vi "8-Axis (Manual).vi"() -> ()   [LabVIEW 2014]
uses:
  EMC API/EMC_Typedef_Motor_Parameters.ctl
  Typedef/Typedef_Motor_Action.ctl
  <vilib>/Motion/Express/_s/nimc.ex.power.power.axis.vi
  <vilib>/Motion/Express/_s/nimc.ex.resetPosition.resetPosition.axis.vi
  <vilib>/Motion/Express/_s/nimc.ex.findReferenceMove.startReferenceMove.axis.modeReverseLimit.vi
  <vilib>/Motion/Express/_s/nimc.ex.findReferenceMove.startReferenceMove.axis.modeHome.vi
  <vilib>/Motion/Express/_s/nimc.ex.findReferenceMove.startReferenceMove.axis.modeForwardLimit.vi
  <vilib>/Motion/Express/_s/nimc.ex.read.readTrajectoryData.axis.vi
  <vilib>/Motion/Express/_s/nimc.ex.read.readMotionIO.axis.vi
  <vilib>/Motion/BlockNode/FB.NIMotion.xnode
  Functional_Global/Typedef_FPGA_Interface_Action.ctl
  <vilib>/Motion/Express/_s/nimc.ex.clearFaults.clearFaults.axis.vi
panel:
  in  "velocity":dbl=1000.0
  in  "position[]":dbl[](array[numeric])=[5000.0, 5000.0, 5000.0, 5000.0, 5000.0, 5000.0, 5000.0, 5000.0]
  in  "resource":refnum<k21>="Axis 1"
  out "home active":bool
  out "rev. limit active":bool
  out "fwd. limit active":bool
  out "XY Graph":cluster{"X Array":dbl[], "Y Array":dbl[]}(graph)
  in  "interval":dbl=0.01 format="%#_13g"
  in  "Gear in/out":enum16{"Gear in", "Gear out"}(ring)
  in  "denominator":i32=1
  in  "numerator":i32=1
  in  "Master Axis":T1(ring)
  out "Array":dbl[](array[knob]) scale=0.0..1600.0
  in  "Clear Errors":bool
  in  "Command":T2
  in  "Motion Parameters":T3={"position"=1000.0, "velocity"=1000.0, "acceleration"=10000.0, "deceleration"=10000.0, "accel. jerk"=10000.0, "decel. jerk"=10000.0}
  in  "Axis Index":T1(ring)
  out "error":errorcluster
  out "Numeric":i32
  in  "Stop all motors":bool
  in  "Execute Command":bool
  in  "stop":bool
  out "Axis Velocities":T4(graph)
  out "Axis Positions":T4(graph)
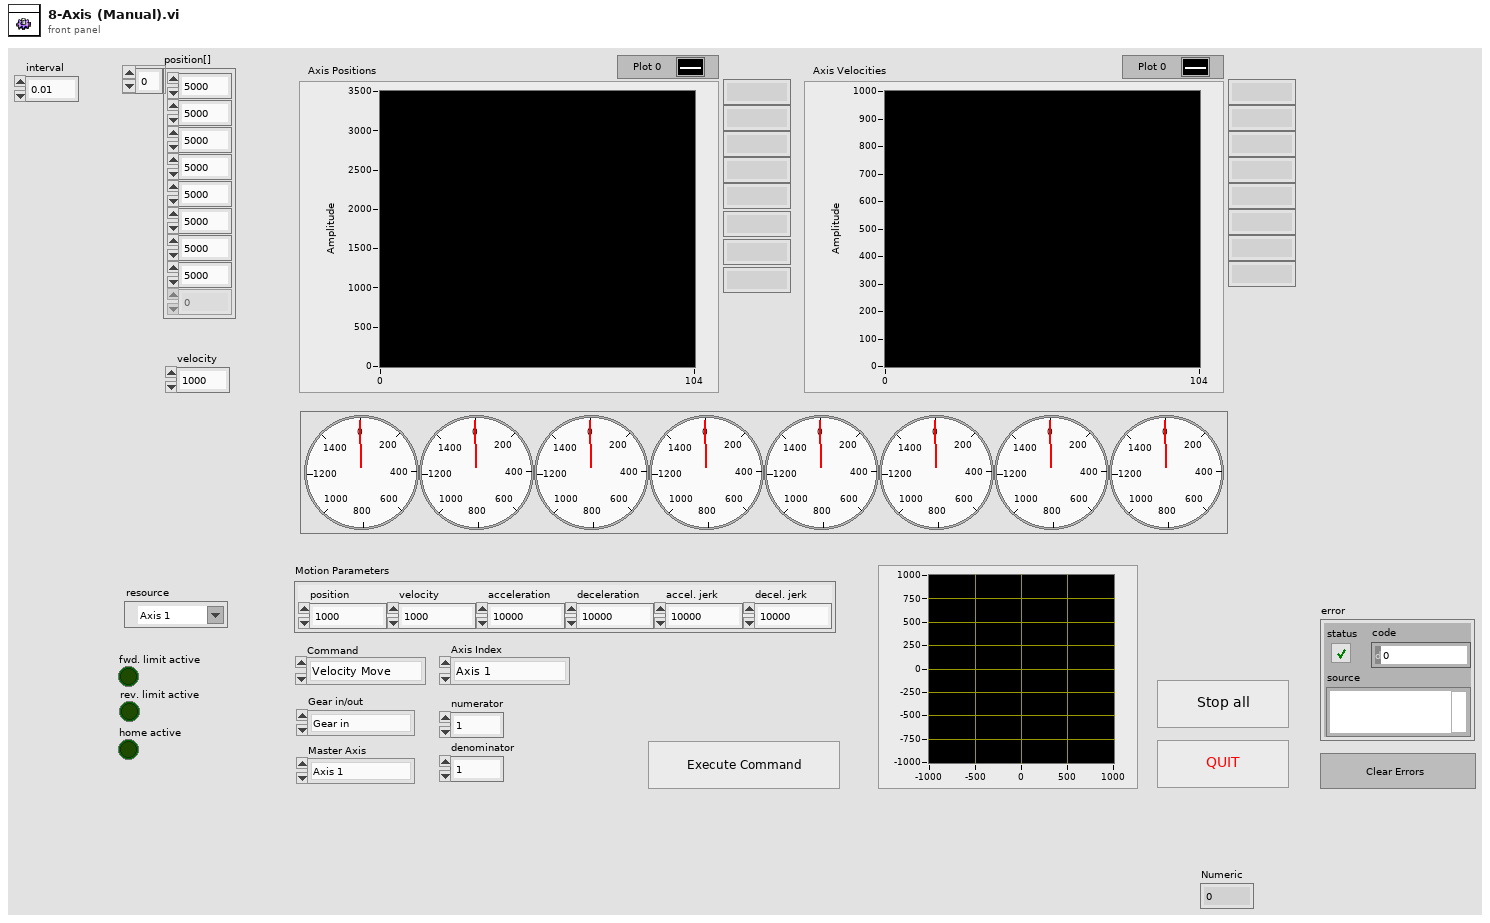
[diagram p1: front panel]
types:
  T1 = enum16{"Axis 1", "Axis 2", "Axis 3", "Axis 4", "Axis 5", "Axis 6", "Axis 7", "Axis 8"}
  T2 = typedef "Typedef_Motor_Action.ctl" = enum16{"Velocity Move", "REL Pos Move", "ABS Pos Move", "Stop", "Reset Position", "Coordinate_move", "Contour_move", "Gearing", "Find Fwd Limit", "Find Rev Limit", "Find Home"}
  T3 = typedef "EMC_Typedef_Motor_Parameters.ctl" = cluster{"position":dbl, "velocity":dbl, "acceleration":dbl, "deceleration":dbl, "accel. jerk":dbl, "decel. jerk":dbl}
  T4 = cluster{"[0]":dbl, "[1]":dbl, "[2]":dbl, "[3]":dbl, "[4]":dbl, "[5]":dbl, "[6]":dbl, "[7]":dbl}
  T5 = typedef "Typedef_FPGA_Interface_Action.ctl" = enum16{"Initialize FPGA", "Get FPGA Reference", "Close FPGA"}
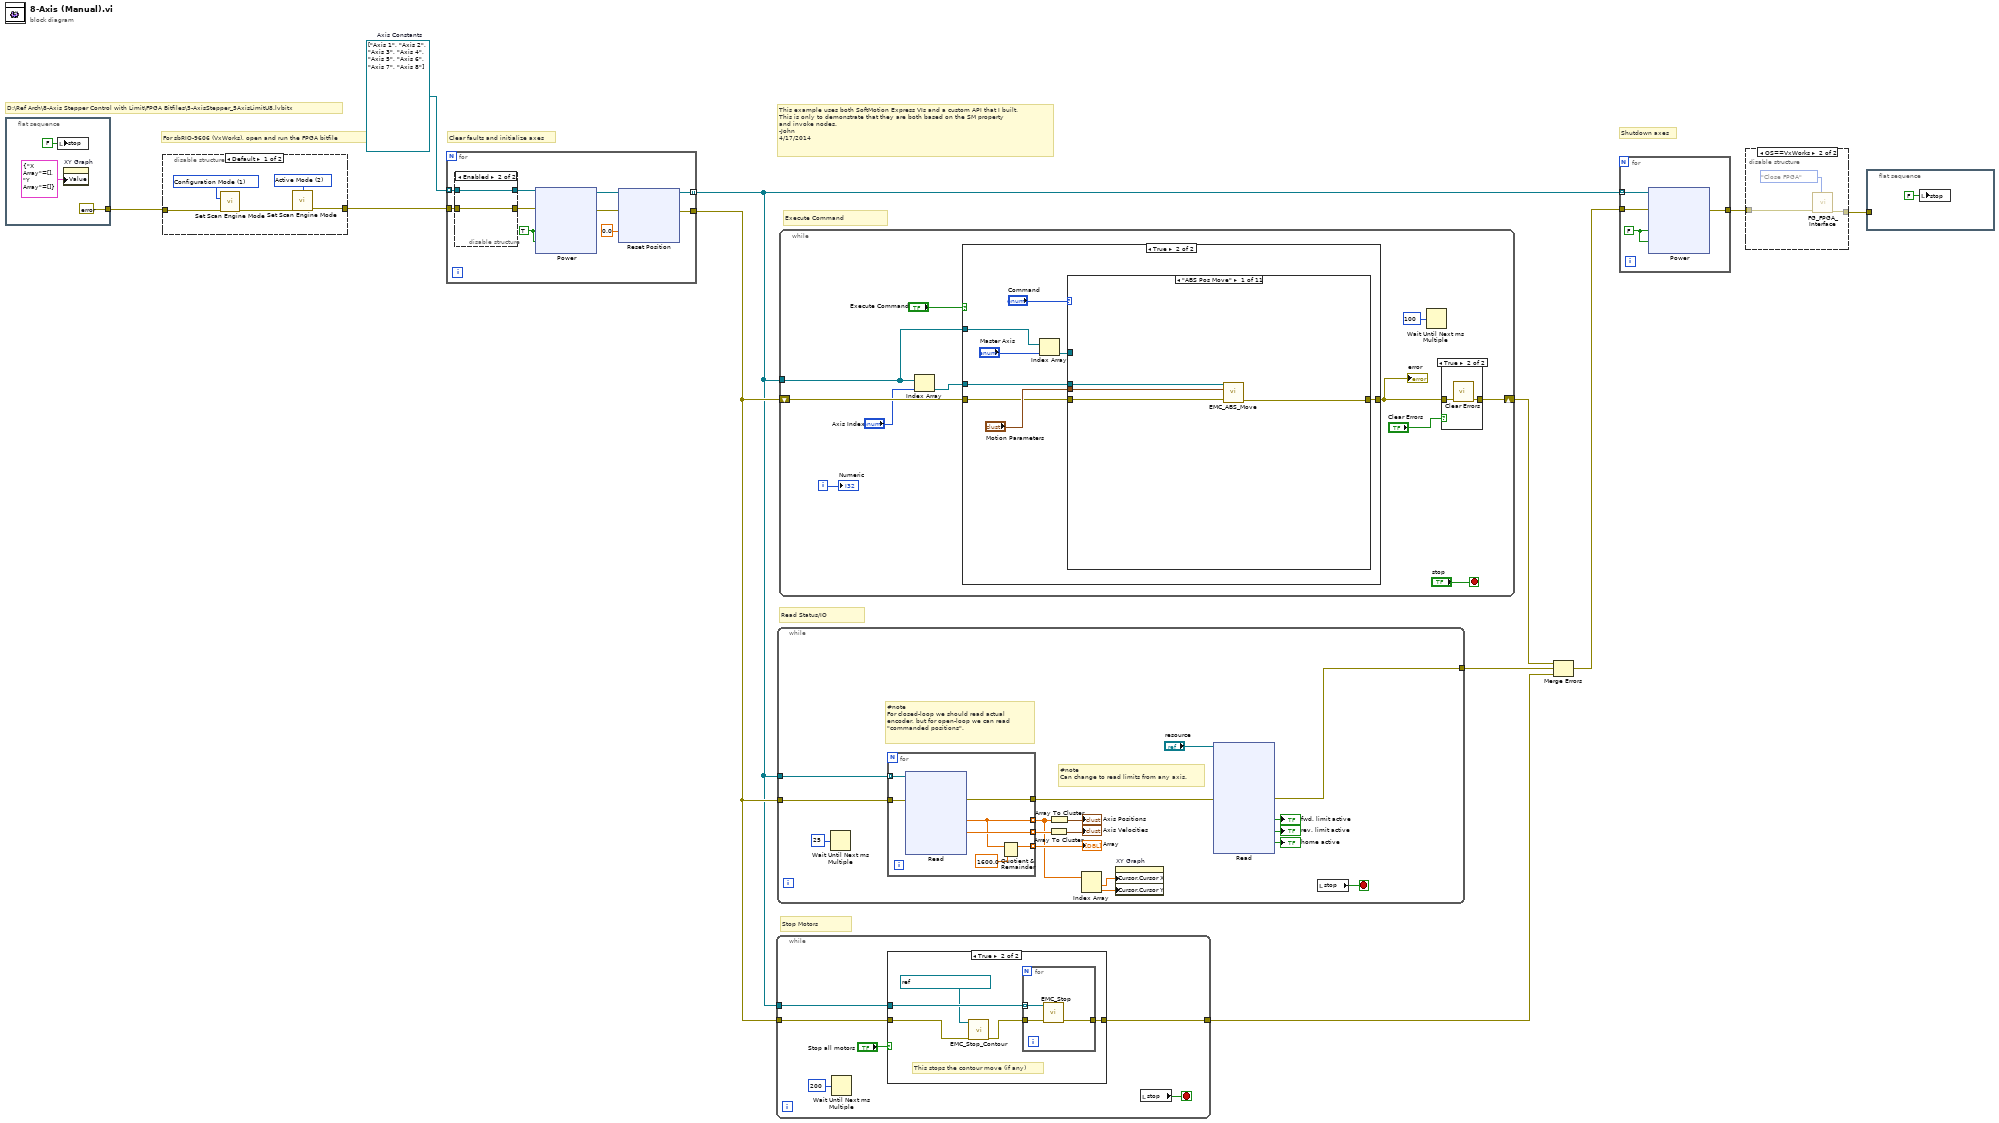
[diagram p0: block diagram]
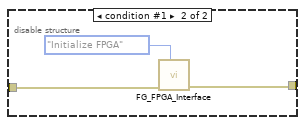
[diagram p3: hidden frame]
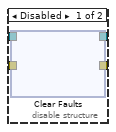
[diagram p4: hidden frame]
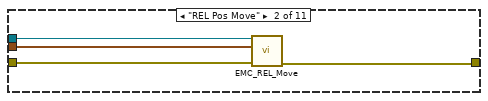
[diagram p8: hidden frame]
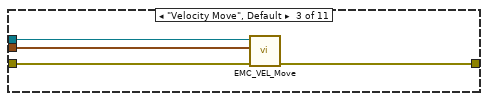
[diagram p9: hidden frame]
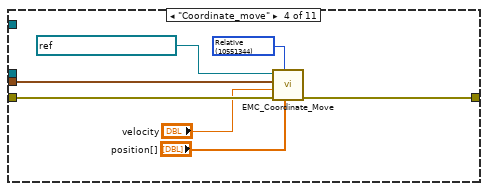
[diagram p10: hidden frame]
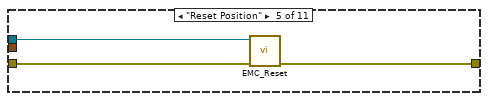
[diagram p11: hidden frame]
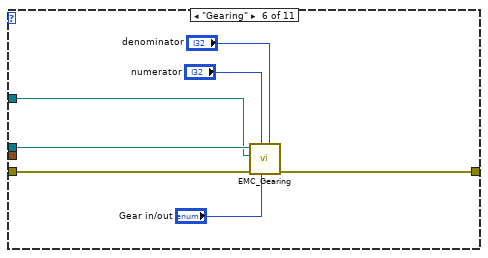
[diagram p12: hidden frame]
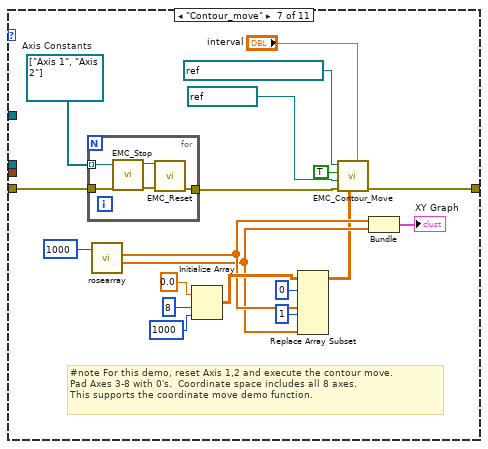
[diagram p13: hidden frame]
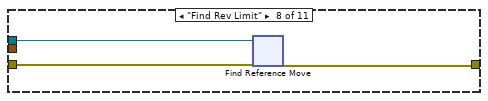
[diagram p14: hidden frame]
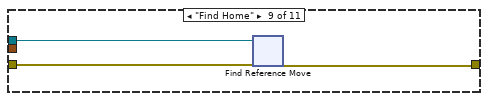
[diagram p15: hidden frame]
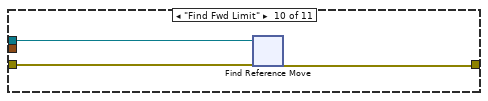
[diagram p16: hidden frame]
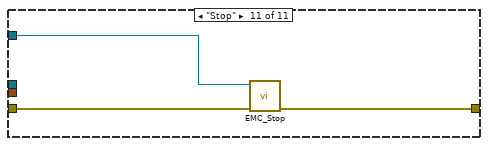
[diagram p17: hidden frame]
diagram:
  w10 = refnum<k21>[] ["Axis 1", "Axis 2", "Axis 3", "Axis 4", "Axis 5", "Axis 6", "Axis 7", "Axis 8"]  # Axis Constants
  # "For sbRIO-9606 (VxWorks), open and run the FPGA bitfile"
  # "D:\\Ref Arch\\8-Axis Stepper Control with Limit\\FPGA Bitfiles\\5-AxisStepper_5AxisLimitU8.lvbitx"
  # "Clear faults and initialize axes"
  # "This example uses both SoftMotion Express VIs and a custom API that I built.\nThis is only to demonstrate that they are both based on the SM property\nand invoke nodes. \n-John\n4/17/2014"
  # "Shutdown axes"
  # "Execute Command"
  # "Read Status/IO"
  # "Stop Motors"
  n1 = flat-sequence {
    tunnel: [errorcluster {"status"=FALSE, "code"=0, "source"=""} ("error in (no error)")] -> w7
    frame #0 {
      n2 = local write "stop"(FALSE ("stop")) -> ()
      n3 = property on="XY Graph" class="XYGraph (strict)"("Value"=cluster{"X Array":dbl[], "Y Array":dbl[]} {"X Array"=[], "Y Array"=[]} ("XY Graph")) -> ()  [unwired: 2 in, 2 out]
    }
  }
  n4 = disable-structure shown="Default" {
    disable-tunnel: [w19 w20] -> w4
    disable-tunnel: w7 -> [w18 w21]
    frame condition #0 (active) {
      w15 = 1 items=["Configuration Mode"=1, "Active Mode"=2] ("mode (Active Mode)")
      w16 = 2 items=["Configuration Mode"=1, "Active Mode"=2] ("mode (Active Mode)")
      n5 = call <vilib>:"Set Scan Engine Mode.vi"("mode (Active Mode)"=w15, "error in (no error)"=w18) -> ("error out"=w17:errorcluster)  [unwired: 13 in]
      n6 = call <vilib>:"Set Scan Engine Mode.vi"("mode (Active Mode)"=w16, "error in (no error)"=w17) -> ("error out"=w19:errorcluster)  [unwired: 13 in]
    }
    frame condition #1 {
      n7 = call "FG_FPGA_Interface.vi"("Action"=Typedef_FPGA_Interface_Action."Initialize FPGA", "error in"=w21) -> ("error out"=w20:errorcluster)  [unwired: 9 in]
    }
  }
  n8 = for {
    tunnel: w10 -> [w26] mode=indexing
    tunnel: w4 -> [w25]
    tunnel: [w28] -> w3
    tunnel: [w27] -> w1 mode=indexing
    w32 = TRUE ("enable axis")
    n9 = disable-structure shown="Enabled" {
      disable-tunnel: w26 -> [w36 w42]
      disable-tunnel: w25 -> [w35 w41]
      disable-tunnel: [w34 w42] -> w24
      disable-tunnel: [w33 w41] -> w23
      frame Disabled {
        n10 = xnode ("Clear Faults")("resource"=w36, "error in"=w35) -> ("resource out"=w34:refnum<k21>, "error out"=w33:errorcluster)
      }
      frame Enabled {
      }
    }
    n11 = xnode ("Power")("enable axis"=w32, "enable drive"=w32, "resource"=w24, "error in"=w23) -> ("resource out"=w31:refnum<k21>, "error out"=w30:errorcluster)
    n12 = xnode ("Reset Position")("position"=0.0, "resource"=w31, "error in"=w30) -> ("resource out"=w27:refnum<k21>, "error out"=w28:errorcluster)
  }
  n13 = while {
    tunnel: w3 -> [w62]
    tunnel: w1 -> [w60]
    tunnel: [w58] -> w11
    stop <- w63 stop-if-true
    n14 = Wait Until Next ms Multiple(millisecond multiple=u32 200) -> ()  [unwired: 1 out]
    n15 = case shown="True" "Stop all motors" {
      tunnel: w62 -> [w64 w67]
      tunnel: [w64 w69] -> w58
      tunnel: w60 -> [_ w68]
      frame False {
      }
      frame True {
        # "This stops the contour move (if any)"
        n16 = call "EMC_Stop_Contour.vi"("error in (no error)"=w67, "coordinate"=refnum<k21> "Coordinate Space 1") -> ("error out"=w65:errorcluster)  [unwired: 9 in]
        n17 = for {
          tunnel: w65 -> [w72]
          tunnel: w68 -> [w70] mode=indexing
          tunnel: [w71] -> w69
          n18 = call "EMC_Stop.vi"("error in (no error)"=w72, "axis"=w70) -> ("error out"=w71:errorcluster)  [unwired: 8 in, 1 out]
        }
      }
    }
    n19 = local read "stop"() -> (w63:bool)
  }
  n20 = while {
    tunnel: w3 -> [w85]
    tunnel: w1 -> [w84]
    tunnel: [w73] -> w9
    stop <- w89 stop-if-true
    # "#note \nCan change to read limits from any axis."
    # "#note \nFor closed-loop we should read actual \nencoder, but for open-loop we can read\n\"commanded positions\"."
    n21 = Wait Until Next ms Multiple(millisecond multiple=u32 25) -> ()  [unwired: 1 out]
    n22 = for {
      tunnel: [w124] -> w75
      tunnel: [w119] -> w82 mode=indexing
      tunnel: [w123] -> w88 mode=indexing
      tunnel: w85 -> [w122]
      tunnel: w84 -> [w121] mode=indexing
      tunnel: [w118] -> w83 mode=indexing
      n23 = xnode ("Read")("resource"=w121, "error in"=w122) -> ("commanded position"=w119:dbl, "commanded vel."=w123:dbl, "error out"=w124:errorcluster)  [unwired: 2 out]
      n24 = Quotient & Remainder(x=w119, y=1600.0) -> (x-y*floor(x/y)=w118:dbl)  [unwired: 1 out]
    }
    "Array" <- w83
    n25 = Array To Cluster(array=w88) -> (cluster=→"Axis Velocities":T4)
    n26 = Array To Cluster(array=w82) -> (cluster=→"Axis Positions":T4)
    n27 = Index Array(array=w82) -> (element #1=w81:dbl, element #2=w80:dbl)  [unwired: 2 in]
    n28 = property on="XY Graph" class="XYGraph (strict)"("Cursor.Cursor X"=w81, "Cursor.Cursor Y"=w80) -> ()  [unwired: 2 in, 2 out]
    n29 = xnode ("Read")("resource"="resource", "error in"=w75) -> ("fwd. limit active"=→"fwd. limit active":bool, "rev. limit active"=→"rev. limit active":bool, "home active"=→"home active":bool, "error out"=w73:errorcluster)  [unwired: 6 out]
    n30 = local read "stop"() -> (w89:bool)
  }
  n31 = while {
    tunnel: w1 -> [w132]
    shift-right: [w133] -> w6
    shift-left: w3 -> [w137]
    i -> [w142]
    stop <- "stop" stop-if-true
    n32 = Index Array(array=w132, index="Axis Index") -> (element=w138:refnum<k21>)
    n33 = case shown="True" "Execute Command" {
      tunnel: w137 -> [w146 w153]
      tunnel: w138 -> [_ w152]
      tunnel: [w146 w151] -> w134
      tunnel: w132 -> [_ w148]
      frame False {
      }
      frame True {
        n34 = Index Array(array=w148, index="Master Axis") -> (element=w147:refnum<k21>)
        n35 = case shown="\"ABS Pos Move\"" "Command" {
          tunnel: "Motion Parameters" -> [w155 w159 w166 w167 _ _ _ _ _ _ _]
          tunnel: w153 -> [w158 w162 w165 w173 w176 w183 w195 w209 w228 w249 w269]
          tunnel: w152 -> [w156 w160 w164 _ w175 w182 _ w208 w227 w248 _]
          tunnel: [w157 w161 w163 w172 w174 w181 w202 w210 w229 w250 w268] -> w151
          tunnel: w147 -> [_ _ _ _ _ w177 _ _ _ _ w267]
          frame "ABS Pos Move" {
            n36 = call "EMC_ABS_Move.vi"("error in (no error)"=w158, "Motion Parameters"=w155, "axis"=w156) -> ("error out"=w157:errorcluster)  [unwired: 8 in]
          }
          frame "REL Pos Move" {
            n37 = call "EMC_REL_Move.vi"("error in (no error)"=w162, "Motion Parameters"=w159, "axis"=w160) -> ("error out"=w161:errorcluster)  [unwired: 8 in]
          }
          frame "Velocity Move", Default {
            n38 = call "EMC_VEL_Move.vi"("error in (no error)"=w165, "Motion Parameters"=w166, "axis"=w164) -> ("error out"=w163:errorcluster)  [unwired: 8 in]
          }
          frame "Coordinate_move" {
            w170 = 10551344 items=["Relative"=10551344, "Absolute"=10551337, "Relative To Capture"=10551345, "Velocity"=10551346, "Polyline"=11600101] ("line move mode")
            n39 = call "EMC_Coordinate_Move.vi"("position[]"="position[]", "line move mode"=w170, "error in (no error)"=w173, "velocity"="velocity", "Motion Parameters"=w167, "resource"=refnum<k21> "Coordinate Space 1") -> ("error out"=w172:errorcluster)  [unwired: 5 in]
          }
          frame "Reset Position" {
            n40 = call "EMC_Reset.vi"("error in (no error)"=w176, "axis"=w175) -> ("error out"=w174:errorcluster)  [unwired: 9 in]
          }
          frame "Gearing" {
            n41 = call "EMC_Gearing.vi"("denominator"="denominator", "Gear in/out"="Gear in/out", "numerator"="numerator", "error in (no error)"=w183, "master axis"=w177, "axis"=w182) -> ("error out"=w181:errorcluster)  [unwired: 5 in]
          }
          frame "Contour_move" {
            w193 = refnum<k21>[] ["Axis 1", "Axis 2"]  # Axis Constants
            # "#note For this demo, reset Axis 1,2 and execute the contour move.\nPad Axes 3-8 with 0's.  Coordinate space includes all 8 axes.\nThis supports the coordinate move demo function."
            n42 = for {
              tunnel: w195 -> [w206]
              tunnel: [w207] -> w194
              tunnel: w193 -> [w204] mode=indexing
              n43 = call "EMC_Stop.vi"("error in (no error)"=w206, "axis"=w204) -> ("error out"=w205:errorcluster, "axis out"=w203:refnum<k21>)  [unwired: 8 in]
              n44 = call "EMC_Reset.vi"("error in (no error)"=w205, "axis"=w203) -> ("error out"=w207:errorcluster)  [unwired: 9 in]
            }
            n45 = call "rosearray.vi"("Iterations"=u32 1000) -> ("Y Array"=w185:dbl[], "X Array"=w186:dbl[])  [unwired: 5 in, 1 out]
            n46 = Initialize Array(0.0 ("element"), 8 ("dimension size"), 1000 ("dimension size")) -> (w190:dbl[][])
            n47 = Replace Array Subset(array=w190, new element #1=w186, index (row) #1=0 ("index (row)"), new element #2=w185, index (row) #2=1 ("index (row)")) -> (w184:dbl[][])  [unwired: 2 in]
            n48 = call "EMC_Contour_Move.vi"("interval"="interval", "points[][]"=w184, "error in (no error)"=w194, "table"=refnum<k21> "Table 1" ("resource"), "overwrite"=TRUE, "coordinate"=refnum<k21> "Coordinate Space 1" ("resource")) -> ("error out"=w202:errorcluster)  [unwired: 5 in]
            n49 = Bundle("X Array"=w186, "Y Array"=w185) -> (→"XY Graph":cluster{"X Array":dbl[], "Y Array":dbl[]})  [unwired: 1 in]
          }
          frame "Find Rev Limit" {
            n50 = xnode "Find Reference Move"("resource"=w208, "error in"=w209) -> ("error out"=w210:errorcluster)  [unwired: 9 in, 2 out]
          }
          frame "Find Home" {
            n51 = xnode "Find Reference Move"("resource"=w227, "error in"=w228) -> ("error out"=w229:errorcluster)  [unwired: 11 in, 2 out]
          }
          frame "Find Fwd Limit" {
            n52 = xnode "Find Reference Move"("resource"=w248, "error in"=w249) -> ("error out"=w250:errorcluster)  [unwired: 9 in, 2 out]
          }
          frame "Stop" {
            n53 = call "EMC_Stop.vi"("error in (no error)"=w269, "axis"=w267) -> ("error out"=w268:errorcluster)  [unwired: 8 in, 1 out]
          }
        }
      }
    }
    "error" <- w134
    n54 = Wait Until Next ms Multiple(millisecond multiple=u32 100) -> ()  [unwired: 1 out]
    n55 = case shown="True" "Clear Errors" {
      tunnel: w134 -> [w143 w145]
      tunnel: [w143 w144] -> w133
      frame False {
      }
      frame True {
        n56 = call <vilib>:"Clear Errors.vi"("error in (no error)"=w145) -> ("error out"=w144:errorcluster)  [unwired: 5 in, 1 out]
      }
    }
    "Numeric" <- w142
  }
  n57 = Merge Errors(w6, w9, w11) -> (w2:errorcluster)
  n58 = for {
    tunnel: w1 -> [w273] mode=indexing
    tunnel: [w271] -> w5
    tunnel: w2 -> [w270]
    w272 = FALSE ("enable axis")
    n59 = xnode ("Power")("enable axis"=w272, "enable drive"=w272, "resource"=w273, "error in"=w270) -> ("error out"=w271:errorcluster)  [unwired: 1 out]
  }
  n60 = disable-structure shown="OS==VxWorks" {
    disable-tunnel: w5 -> [w284 w286]
    disable-tunnel: [w284 w285] -> w8
    frame condition #0 (active) {
    }
    frame condition #1 {
      n61 = call "FG_FPGA_Interface.vi"("Action"=Typedef_FPGA_Interface_Action."Close FPGA", "error in"=w286) -> ("error out"=w285:errorcluster)  [unwired: 9 in]
    }
  }
  n62 = flat-sequence {
    tunnel: w8 -> [_]
    frame #0 {
      n63 = local write "stop"(FALSE ("stop")) -> ()
    }
  }
